vi "Facade.vi"(0 "Data In":T4, 2 "Display State In":T2, 3 "Container State":T3) -> (6 "Data Out":T4, 7 "Display State Out":T2, 8 "Action":T1)   [LabVIEW 2021, in "myRIO Choice Button.xctl"]
uses:
  <vilib>/myRIO/Common/Instrument Driver Framework/Utilities/xctls/myRIO Choice Button/myRIO Choice Button.xctl
  <vilib>/myRIO/Common/Instrument Driver Framework/Utilities/xctls/myRIO Choice Button/Data.ctl
  <vilib>/_xctls/Container State.ctl
  <vilib>/myRIO/Common/Instrument Driver Framework/Utilities/xctls/myRIO Choice Button/State.ctl
  <vilib>/_xctls/Action.ctl
  <vilib>/Utility/miscctls.llb/LVPositionTypeDef.ctl
  <vilib>/picture/picture.llb/imagedata.ctl
  <vilib>/_xctls/XControlSupport.lvlib
panel:
  out "Button Square":picture
  out "Explanation":string
  out "Title":string
  out "Glyph":picture
  out "Background":picture
types:
  T1 = typedef "XControlSupport.lvlib/Action.ctl" = cluster{"Data Changed?":bool, "State Changed?":bool, "Action Name":string}
  T2 = typedef "myRIO Choice Button.xctl/State.ctl" = cluster{"Title":string, "Explanation":string, "Mouse Enter Glyph":picture, "Mouse Down Glyph":picture, "Mouse Leave Glyph":picture, "Mouse Enter Background":picture, "Mouse Down Background":picture, "Mouse Leave Background":picture, "Button Mode":i32, "Button Square Frame":picture, "Disabled&GrayedOut":bool}
  T3 = typedef "XControlSupport.lvlib/Container State.ctl" = cluster{"Indicator?":bool, "Run Mode?":bool, " Refnum":refnum<vi>}
  T4 = typedef "myRIO Choice Button.xctl/Data.ctl" = bool
  T5 = typedef "LVPositionTypeDef.ctl" = cluster{"Left":i32, "Top":i32}
  T6 = enum8{"Enabled", "Disabled", "Disabled and Grayed Out"}
  T7 = typedef "imagedata.ctl" = cluster{"image type":i32, "image depth":i32, "image":u8[], "mask":u8[], "colors":u32[], "Rectangle":cluster{"left":i16, "top":i16, "right":i16, "bottom":i16}}
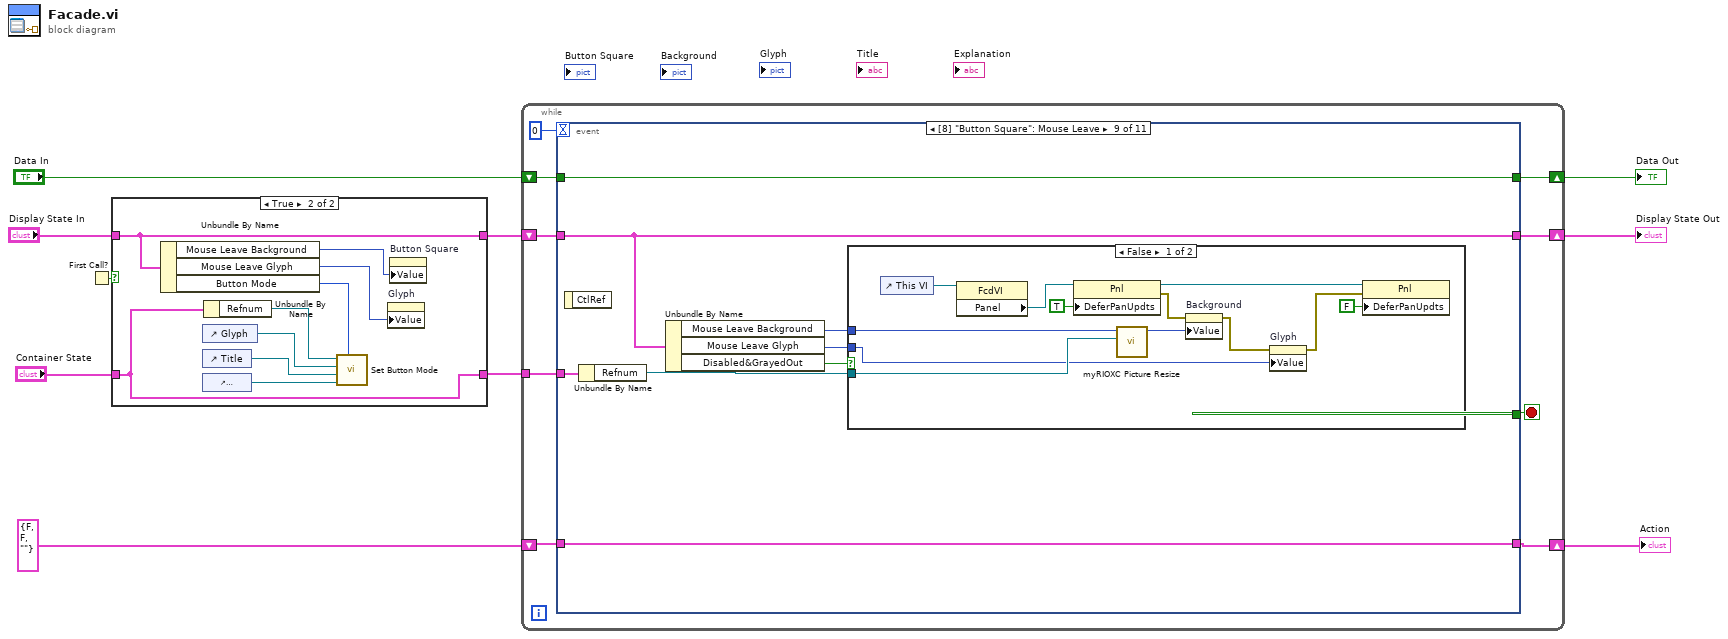
[diagram p0: block diagram]
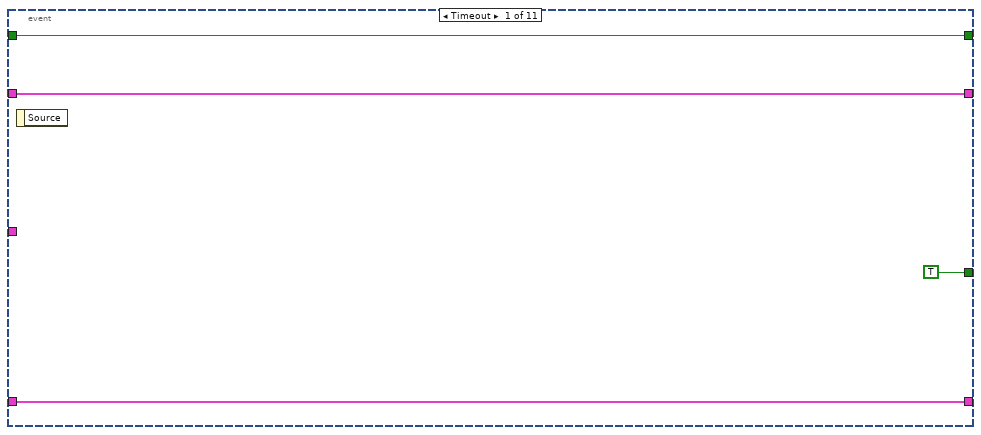
[diagram p3: hidden frame]
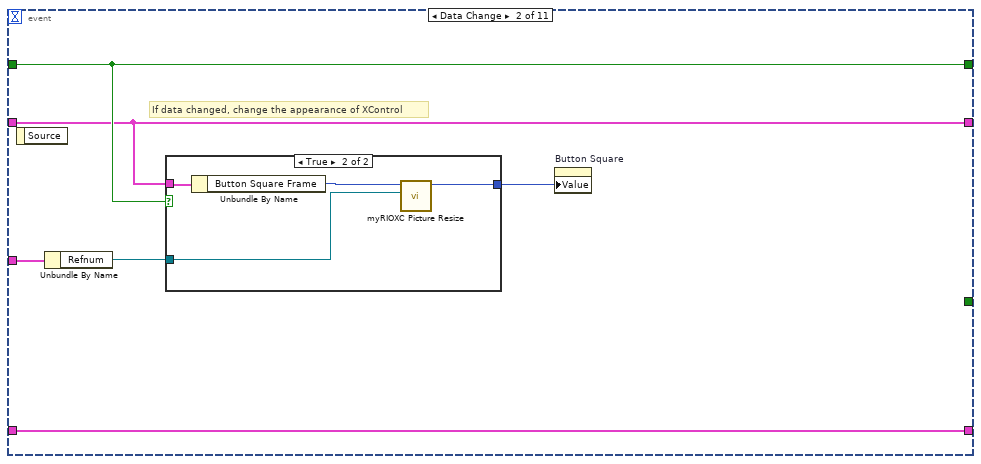
[diagram p4: hidden frame]
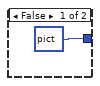
[diagram p5: hidden frame]
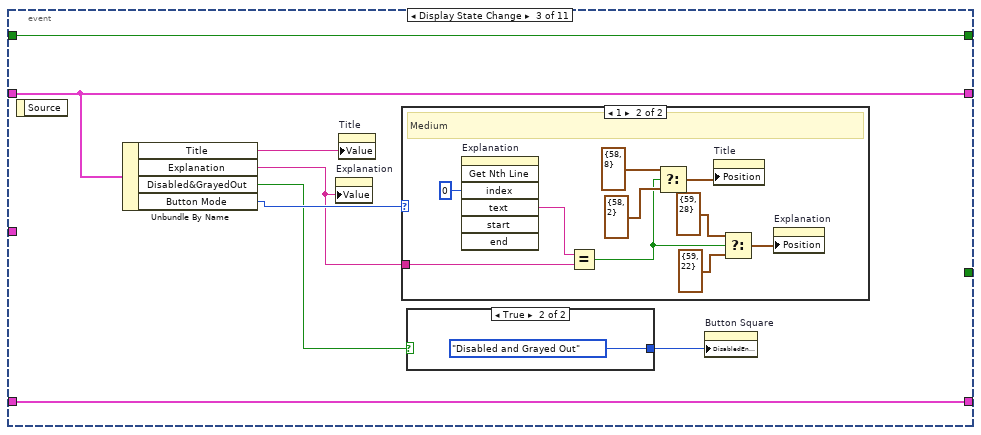
[diagram p6: hidden frame]
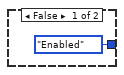
[diagram p8: hidden frame]
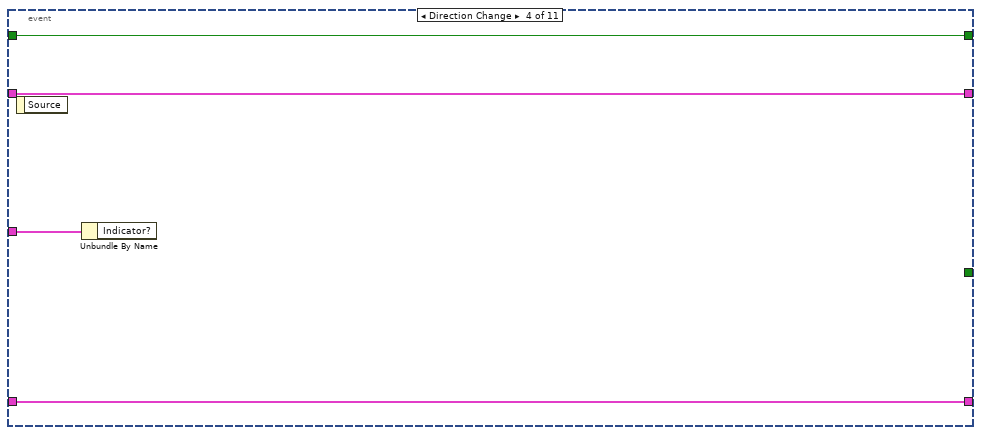
[diagram p9: hidden frame]
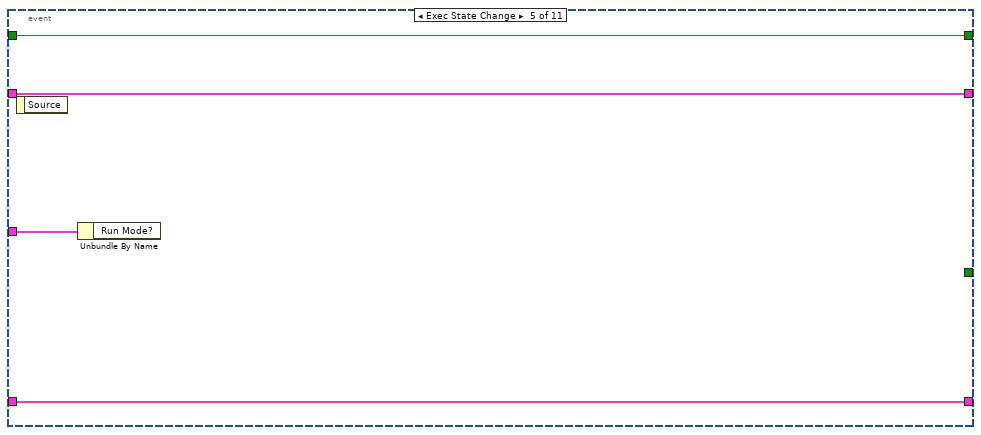
[diagram p10: hidden frame]
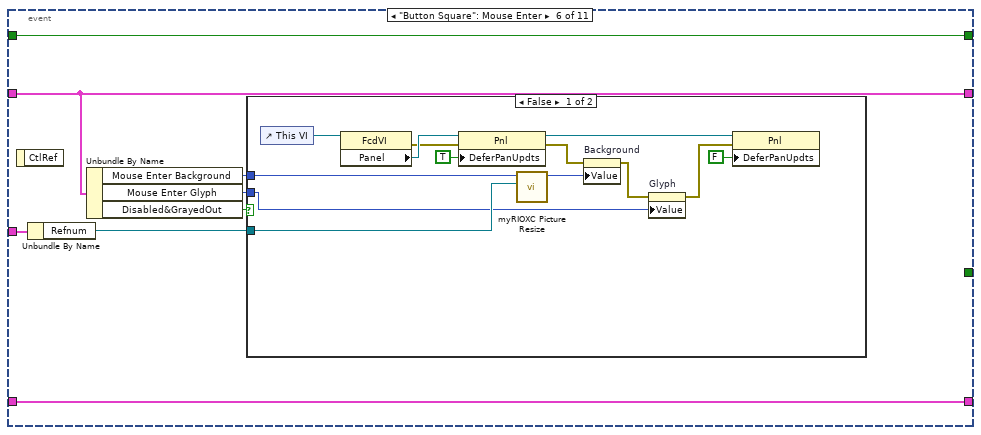
[diagram p11: hidden frame]
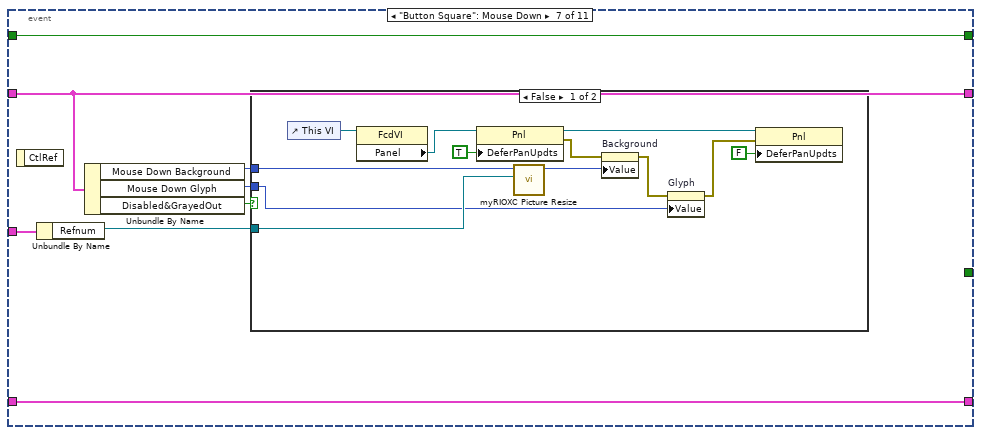
[diagram p13: hidden frame]
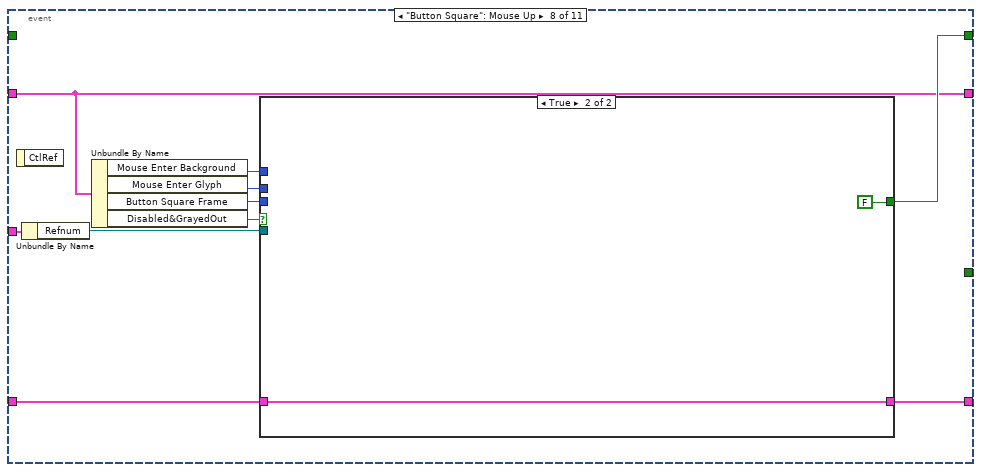
[diagram p15: hidden frame]
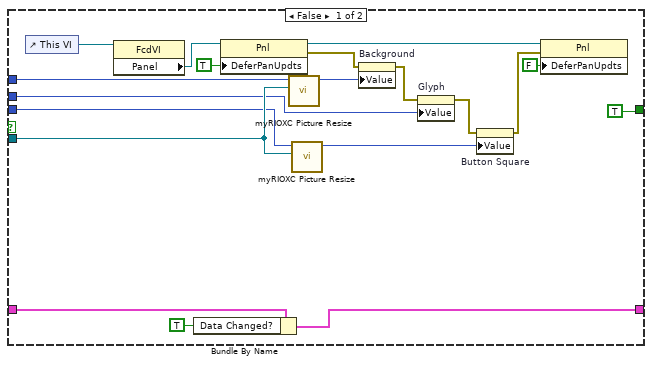
[diagram p16: hidden frame]
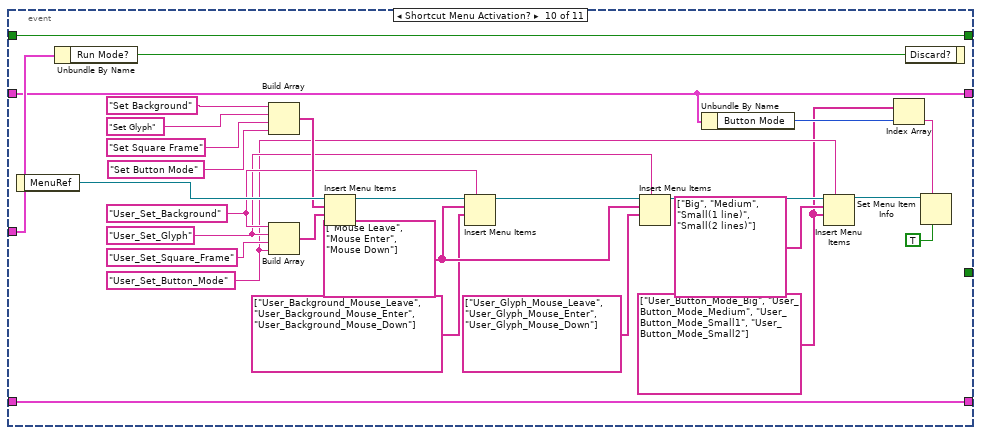
[diagram p18: hidden frame]
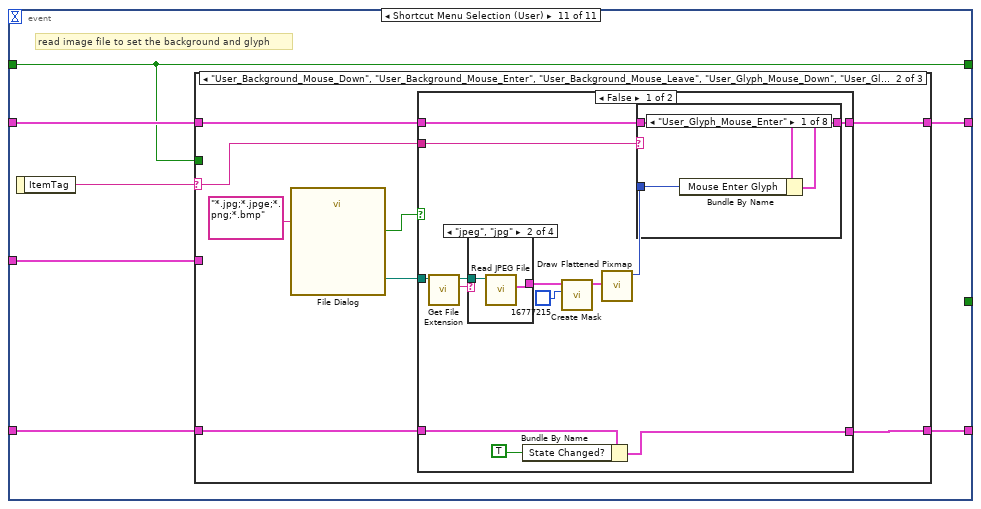
[diagram p19: hidden frame]
diagram:
  n1 = First Call?() -> (First Call?: T/F=w3:bool)
  n2 = case shown="True" w3 {
    tunnel: [w12 w19] -> w5
    tunnel: "Display State In" -> [w12 w19]
    tunnel: "Container State" -> [w11 w18]
    tunnel: [w11 w18] -> w1
    frame False {
    }
    frame True {
      n3 = Unbundle By Name(w19) -> ("Mouse Leave Background"=w20:picture, "Mouse Leave Glyph"=w21:picture, "Button Mode"=w17:i32)
      n4 = control-ref of="Glyph"() -> (w15:refnum<vi>)
      n5 = control-ref of="Title"() -> (w14:refnum<vi>)
      n6 = control-ref of="Explanation"() -> (w13:refnum<vi>)
      n7 = Unbundle By Name(w18) -> ("Refnum"=w16:refnum<vi>)
      n8 = call <vilib>:"Set Button Mode.vi"("Button Mode"=w17, "Explanation"=w13, "Title"=w14, "Glyph"=w15, "Container Reference"=w16) -> ()  [unwired: 7 in]
      n9 = property on="Glyph" class="Pict"("Value"=w21) -> ()  [unwired: 2 in, 2 out]
      n10 = property on="Button Square" class="Pict"("Value"=w20) -> ()  [unwired: 2 in, 2 out]
    }
  }
  n11 = while {
    shift-right: [w29] -> w8
    shift-left: w5 -> [w30]
    tunnel: w1 -> [w27]
    shift-right: [w25] -> w10
    shift-left: "Data In" -> [w26]
    shift-right: [w23] -> w7
    shift-left: T1 {"Data Changed?"=FALSE, "State Changed?"=FALSE, "Action Name"=""} ("Action") -> [w24]
    stop <- w28 stop-if-true
    n12 = event shown="[8] \"Button Square\": Mouse Leave" {
      selector: _ -> [_ _ _ _ _ _ _ _ _ _ _]
      dyn-events: _ -> [_ _ _ _ _ _ _ _ _ _ _]
      timeout: 0 -> [_ _ _ _ _ _ _ _ _ _ _]
      tunnel: w30 -> [w32 w37 w53 w68 w72 w77 w98 w120 w149 w171 w200]
      tunnel: [w32 w37 w53 w68 w72 w77 w98 w120 w149 w171 w199] -> w29
      tunnel: [TRUE _ _ _ _ _ _ _ _ _ _] -> w28
      tunnel: w27 -> [_ w36 _ w69 w73 w79 w100 w122 w151 w180 w195]
      tunnel: w26 -> [w31 w39 w50 w67 w71 w80 w101 _ w153 w193 w194]
      tunnel: [w31 w39 w50 w67 w71 w80 w101 w121 w153 w193 w194] -> w25
      tunnel: [w33 w40 w52 w66 w70 w81 w102 w123 w152 w192 w198] -> w23
      tunnel: w24 -> [w33 w40 w52 w66 w70 w81 w102 w124 w152 w192 w197]
      event Timeout {
        n13 = event-data() -> ()  [unwired: 1 in, 1 out]
      }
      event Data Change {
        # "If data changed, change the appearance of XControl"
        n14 = event-data() -> ()  [unwired: 1 in, 1 out]
        n15 = Unbundle By Name(w36) -> ("Refnum"=w35:refnum<vi>)
        n16 = case shown="True" w39 {
          tunnel: [picture data[5B] ("new picture") w43] -> w38
          tunnel: w37 -> [_ w45]
          tunnel: w35 -> [_ w42]
          frame False {
          }
          frame True {
            n17 = Unbundle By Name(w45) -> ("Button Square Frame"=w44:picture)
            n18 = call <vilib>:"myRIOXC Picture Resize.vi"("XCtrl Reference"=w42, "picture"=w44) -> ("new picture"=w43:picture)  [unwired: 9 in]
          }
        }
        n19 = property on="Button Square" class="Pict"("Value"=w38) -> ()  [unwired: 2 in, 2 out]
      }
      event Display State Change {
        n20 = event-data() -> ()  [unwired: 1 in, 1 out]
        n21 = Unbundle By Name(w53) -> ("Title"=w51:string, "Explanation"=w46:string, "Disabled&GrayedOut"=w47:bool, "Button Mode"=w48:i32)
        n22 = property on="Explanation" class="Str"("Value"=w46) -> ()  [unwired: 2 in, 2 out]
        n23 = property on="Title" class="Str"("Value"=w51) -> ()  [unwired: 2 in, 2 out]
        n24 = case shown="1" w48 {
          tunnel: w46 -> [_ w55]
          frame 0, Default {
            # "Other Modes"
          }
          frame 1 {
            # "Medium"
            n25 = invoke on="Explanation" class="Str" method="Get Nth Line"("index"=u32 0 ("line index")) -> ("text"=w56:string)  [unwired: 6 in, 6 out]
            n26 = Equal?(x=w56, y=w55) -> (x = y?=w54:bool)
            n27 = Select(t=T5 {"Left"=58, "Top"=8} ("Position"), s=w54, f=T5 {"Left"=58, "Top"=2}) -> (s? t:f=w62:T5)
            n28 = property on="Title" class="Str"("Position"=w62) -> ()  [unwired: 2 in, 2 out]
            n29 = Select(t=T5 {"Left"=59, "Top"=28} ("Position"), s=w54, f=T5 {"Left"=59, "Top"=22}) -> (s? t:f=w58:T5)
            n30 = property on="Explanation" class="Str"("Position"=w58) -> ()  [unwired: 2 in, 2 out]
          }
        }
        n31 = case shown="True" w47 {
          tunnel: [T6."Enabled" ("Disabled") T6."Disabled and Grayed Out" ("Disabled")] -> w49
          frame False {
          }
          frame True {
          }
        }
        n32 = property on="Button Square" class="Pict"("DisabledEnum"=w49) -> ()  [unwired: 2 in, 2 out]
      }
      event Direction Change {
        n33 = event-data() -> ()  [unwired: 1 in, 1 out]
        n34 = Unbundle By Name(w69) -> ()  [unwired: 1 out]
      }
      event Exec State Change {
        n35 = event-data() -> ()  [unwired: 1 in, 1 out]
        n36 = Unbundle By Name(w73) -> ()  [unwired: 1 out]
      }
      event "Button Square": Mouse Enter {
        n37 = event-data() -> ()  [unwired: 1 in, 1 out]
        n38 = Unbundle By Name(w79) -> ("Refnum"=w78:refnum<vi>)
        n39 = Unbundle By Name(w77) -> ("Mouse Enter Background"=w75:picture, "Mouse Enter Glyph"=w74:picture, "Disabled&GrayedOut"=w76:bool)
        n40 = case shown="False" w76 {
          tunnel: w78 -> [w93 _]
          tunnel: w75 -> [w83 _]
          tunnel: w74 -> [w82 _]
          frame False {
            n41 = control-ref of="This VI"() -> (w92:refnum<vi>)
            n42 = property class="FcdVI"(reference=w92) -> (error out=w90:errorcluster, "Panel"=w91:refnum<vi>)  [unwired: 1 in, 1 out]
            n43 = property class="Pnl"(reference=w91, error in=w90, "DeferPanUpdts"=TRUE ("Defer Panel Updates")) -> (reference out=w87:refnum<vi>, error out=w88:errorcluster)
            n44 = call <vilib>:"myRIOXC Picture Resize.vi"("XCtrl Reference"=w93, "picture"=w83) -> ("new picture"=w94:picture)  [unwired: 9 in]
            n45 = property on="Background" class="Pict"(error in=w88, "Value"=w94) -> (error out=w86:errorcluster)  [unwired: 1 in, 1 out]
            n46 = property on="Glyph" class="Pict"(error in=w86, "Value"=w82) -> (error out=w85:errorcluster)  [unwired: 1 in, 1 out]
            n47 = property class="Pnl"(reference=w87, error in=w85, "DeferPanUpdts"=FALSE ("Defer Panel Updates")) -> ()  [unwired: 2 out]
          }
          frame True {
          }
        }
      }
      event "Button Square": Mouse Down {
        n48 = event-data() -> ()  [unwired: 1 in, 1 out]
        n49 = Unbundle By Name(w100) -> ("Refnum"=w99:refnum<vi>)
        n50 = Unbundle By Name(w98) -> ("Mouse Down Background"=w95:picture, "Mouse Down Glyph"=w96:picture, "Disabled&GrayedOut"=w97:bool)
        n51 = case shown="False" w97 {
          tunnel: w99 -> [w113 _]
          tunnel: w96 -> [w104 _]
          tunnel: w95 -> [w103 _]
          frame False {
            n52 = control-ref of="This VI"() -> (w112:refnum<vi>)
            n53 = property class="FcdVI"(reference=w112) -> ("Panel"=w107:refnum<vi>)  [unwired: 1 in, 2 out]
            n54 = property class="Pnl"(reference=w107, "DeferPanUpdts"=TRUE ("Defer Panel Updates")) -> (reference out=w111:refnum<vi>, error out=w110:errorcluster)  [unwired: 1 in]
            n55 = call <vilib>:"myRIOXC Picture Resize.vi"("XCtrl Reference"=w113, "picture"=w103) -> ("new picture"=w114:picture)  [unwired: 9 in]
            n56 = property on="Background" class="Pict"(error in=w110, "Value"=w114) -> (error out=w109:errorcluster)  [unwired: 1 in, 1 out]
            n57 = property on="Glyph" class="Pict"(error in=w109, "Value"=w104) -> (error out=w108:errorcluster)  [unwired: 1 in, 1 out]
            n58 = property class="Pnl"(reference=w111, error in=w108, "DeferPanUpdts"=FALSE ("Defer Panel Updates")) -> ()  [unwired: 2 out]
          }
          frame True {
          }
        }
      }
      event "Button Square": Mouse Up {
        n59 = event-data() -> ()  [unwired: 1 in, 1 out]
        n60 = Unbundle By Name(w122) -> ("Refnum"=w119:refnum<vi>)
        n61 = Unbundle By Name(w120) -> ("Mouse Enter Background"=w117:picture, "Mouse Enter Glyph"=w116:picture, "Button Square Frame"=w115:picture, "Disabled&GrayedOut"=w118:bool)
        n62 = case shown="True" w118 {
          tunnel: w124 -> [w143 w145]
          tunnel: [w142 w145] -> w123
          tunnel: [T4 TRUE ("Data In") T4 FALSE ("Data In")] -> w121
          tunnel: w119 -> [w137 _]
          tunnel: w117 -> [w127 _]
          tunnel: w116 -> [w126 _]
          tunnel: w115 -> [w125 _]
          frame False {
            n63 = control-ref of="This VI"() -> (w132:refnum<vi>)
            n64 = property class="FcdVI"(reference=w132) -> ("Panel"=w133:refnum<vi>)  [unwired: 1 in, 2 out]
            n65 = Bundle By Name(cluster=w143, "Data Changed?"=TRUE) -> (w142:T1)
            n66 = property class="Pnl"(reference=w133, "DeferPanUpdts"=TRUE ("Defer Panel Updates")) -> (reference out=w135:refnum<vi>, error out=w131:errorcluster)  [unwired: 1 in]
            n67 = call <vilib>:"myRIOXC Picture Resize.vi"("XCtrl Reference"=w137, "picture"=w127) -> ("new picture"=w139:picture)  [unwired: 9 in]
            n68 = call <vilib>:"myRIOXC Picture Resize.vi"("XCtrl Reference"=w137, "picture"=w125) -> ("new picture"=w138:picture)  [unwired: 9 in]
            n69 = property on="Background" class="Pict"(error in=w131, "Value"=w139) -> (error out=w130:errorcluster)  [unwired: 1 in, 1 out]
            n70 = property on="Glyph" class="Pict"(error in=w130, "Value"=w126) -> (error out=w129:errorcluster)  [unwired: 1 in, 1 out]
            n71 = property on="Button Square" class="Pict"(error in=w129, "Value"=w138) -> (error out=w128:errorcluster)  [unwired: 1 in, 1 out]
            n72 = property class="Pnl"(reference=w135, error in=w128, "DeferPanUpdts"=FALSE ("Defer Panel Updates")) -> ()  [unwired: 2 out]
          }
          frame True {
          }
        }
      }
      event "Button Square": Mouse Leave {
        n73 = event-data() -> ()  [unwired: 1 in, 1 out]
        n74 = Unbundle By Name(w151) -> ("Refnum"=w150:refnum<vi>)
        n75 = Unbundle By Name(w149) -> ("Mouse Leave Background"=w148:picture, "Mouse Leave Glyph"=w147:picture, "Disabled&GrayedOut"=w146:bool)
        n76 = case shown="False" w146 {
          tunnel: w150 -> [w164 _]
          tunnel: w148 -> [w155 _]
          tunnel: w147 -> [w154 _]
          frame False {
            n77 = control-ref of="This VI"() -> (w161:refnum<vi>)
            n78 = property class="FcdVI"(reference=w161) -> ("Panel"=w160:refnum<vi>)  [unwired: 1 in, 2 out]
            n79 = property class="Pnl"(reference=w160, "DeferPanUpdts"=TRUE ("Defer Panel Updates")) -> (reference out=w159:refnum<vi>, error out=w158:errorcluster)  [unwired: 1 in]
            n80 = call <vilib>:"myRIOXC Picture Resize.vi"("XCtrl Reference"=w164, "picture"=w155) -> ("new picture"=w165:picture)  [unwired: 9 in]
            n81 = property on="Background" class="Pict"(error in=w158, "Value"=w165) -> (error out=w157:errorcluster)  [unwired: 1 in, 1 out]
            n82 = property on="Glyph" class="Pict"(error in=w157, "Value"=w154) -> (error out=w156:errorcluster)  [unwired: 1 in, 1 out]
            n83 = property class="Pnl"(reference=w159, error in=w156, "DeferPanUpdts"=FALSE ("Defer Panel Updates")) -> ()  [unwired: 2 out]
          }
          frame True {
          }
        }
      }
      event Shortcut Menu Activation? {
        w166 = string[] ["User_Button_Mode_Big", "User_Button_Mode_Medium", "User_Button_Mode_Small1", "User_Button_Mode_Small2"] ("item tags")
        w173 = "User_Set_Button_Mode"
        w181 = "User_Set_Glyph"
        w182 = "User_Set_Background"
        w186 = string[] ["Mouse Leave", "Mouse Enter", "Mouse Down"] ("item tags")
        n84 = event-data() -> ("MenuRef"=w191:refnum<k9>)  [unwired: 1 in]
        n85 = Unbundle By Name(w180) -> ("Run Mode?"=w179:bool)
        n86 = Build Array("Set Background" ("menu tag"), "Set Glyph" ("menu tag"), "Set Square Frame" ("menu tag"), "Set Button Mode" ("menu tag")) -> (w187:string[])
        n87 = Build Array(w182, w181, "User_Set_Square_Frame", w173) -> (w183:string[])
        n88 = Insert Menu Items(7:w183, 8:w187, 9:w191) -> (3:w178:refnum<k9>)  [unwired: 3 in, 2 out]
        n89 = Insert Menu Items(5:w182, 7:string[] ["User_Background_Mouse_Leave", "User_Background_Mouse_Enter", "User_Background_Mouse_Down"] ("item tags"), 8:w186, 9:w178) -> (3:w190:refnum<k9>)  [unwired: 2 in, 2 out]
        n90 = Insert Menu Items(5:w181, 7:string[] ["User_Glyph_Mouse_Leave", "User_Glyph_Mouse_Enter", "User_Glyph_Mouse_Down"] ("item tags"), 8:w186, 9:w190) -> (3:w174:refnum<k9>)  [unwired: 2 in, 2 out]
        n91 = Unbundle By Name(w171) -> ("Button Mode"=w169:i32)
        n92 = Insert Menu Items(5:w173, 7:w166, 8:string[] ["Big", "Medium", "Small(1 line)", "Small(2 lines)"] ("item tags"), 9:w174) -> (3:w172:refnum<k9>)  [unwired: 2 in, 2 out]
        n93 = Index Array(array=w166, index=w169) -> (element=w168:string)
        n94 = event-data("Discard?"=w179) -> ()  [unwired: 1 in, 1 out]
        n95 = Set Menu Item Info(6:TRUE ("checked"), 7:w168, 11:w172) -> ()  [unwired: 4 in, 2 out]
      }
      event Shortcut Menu Selection (User) {
        # "read image file to set the background and glyph"
        n96 = event-data() -> ("ItemTag"=w196:string)  [unwired: 1 in]
        n97 = case shown="\"User_Background_Mouse_Down\", \"User_Background_Mouse_Enter\", \"User_Background_Mouse_Leave\", \"User_Glyph_Mouse_Down\", \"User_Glyph_Mouse_Enter\", \"User_Glyph_Mouse_Leave\", \"User_Set_Square_Frame\"" w196 {
          selector: w196 -> [_ w203 w258]
          tunnel: w200 -> [w202 w210 w256]
          tunnel: [w202 w209 w262] -> w199
          tunnel: [w201 w208 w265] -> w198
          tunnel: w197 -> [w201 w207 w266]
          tunnel: w195 -> [_ _ w263]
          tunnel: w194 -> [_ _ _]
          frame Default {
          }
          frame "User_Background_Mouse_Down", "User_Background_Mouse_Enter", "User_Background_Mouse_Leave", "User_Glyph_Mouse_Down", "User_Glyph_Mouse_Enter", "User_Glyph_Mouse_Leave", "User_Set_Square_Frame" {
            n98 = call "File Dialog"("pattern (all files)"="*.jpg;*.jpge;*.png;*.bmp") -> ("selected path"=w205:path, "cancelled"=w204:bool)  [unwired: 11 in, 2 out]
            n99 = case shown="False" w204 {
              tunnel: w203 -> [w223 _]
              tunnel: w210 -> [w222 w254]
              tunnel: [w221 w254] -> w209
              tunnel: [w220 w253] -> w208
              tunnel: w207 -> [w218 w253]
              tunnel: w205 -> [w217 _]
              frame False {
                n100 = call <vilib>:"Get File Extension.vi"("file"=w217) -> ("lowercase file extension"=w216:string, "dup file"=w215:path)  [unwired: 6 in, 3 out]
                n101 = case shown="\"jpeg\", \"jpg\"" w216 {
                  tunnel: w215 -> [w225 w227 _ w230]
                  tunnel: [w224 w226 T7 {"image type"=0, "image depth"=0, "image"=[], "mask"=[], "colors"=[], "Rectangle"={"left"=0, "top"=0, "right"=0, "bottom"=0}} ("image data") w229] -> w212
                  frame "bmp" {
                    n102 = call <vilib>:"Read BMP File.vi"("path to BMP file"=w225) -> ("image data"=w224:T7)  [unwired: 8 in, 2 out]
                  }
                  frame "jpeg", "jpg" {
                    n103 = call <vilib>:"Read JPEG File.vi"("path to JPEG file"=w227) -> ("image data"=w226:T7)  [unwired: 8 in, 2 out]
                  }
                  frame Default {
                  }
                  frame "png" {
                    n104 = call <vilib>:"Read PNG File.vi"("path to PNG file"=w230) -> ("image data"=w229:T7)  [unwired: 8 in, 2 out]
                  }
                }
                n105 = Bundle By Name(cluster=w218, "State Changed?"=TRUE) -> (w220:T1)
                n106 = call <vilib>:"Create Mask.vi"("Mask Color (Black)"=u32 16777215, "image data"=w212) -> ("image data"=w211:T7)  [unwired: 9 in]
                n107 = call <vilib>:"Draw Flattened Pixmap.vi"("image data"=w211) -> ("new picture"=w214:picture)  [unwired: 8 in]
                n108 = case shown="\"User_Glyph_Mouse_Enter\"" w223 {
                  tunnel: w222 -> [w232 w234 w237 w240 w243 w246 w249 w252]
                  tunnel: [w233 w234 w236 w239 w242 w245 w248 w251] -> w221
                  tunnel: w214 -> [w231 _ w235 w238 w241 w244 w247 w250]
                  frame "User_Glyph_Mouse_Enter" {
                    n109 = Bundle By Name(cluster=w232, "Mouse Enter Glyph"=w231) -> (w233:T2)
                  }
                  frame Default {
                  }
                  frame "User_Background_Mouse_Enter" {
                    n110 = Bundle By Name(cluster=w237, "Mouse Enter Background"=w235) -> (w236:T2)
                  }
                  frame "User_Background_Mouse_Down" {
                    n111 = Bundle By Name(cluster=w240, "Mouse Down Background"=w238) -> (w239:T2)
                  }
                  frame "User_Background_Mouse_Leave" {
                    n112 = Bundle By Name(cluster=w243, "Mouse Leave Background"=w241) -> (w242:T2)
                  }
                  frame "User_Glyph_Mouse_Down" {
                    n113 = Bundle By Name(cluster=w246, "Mouse Down Glyph"=w244) -> (w245:T2)
                  }
                  frame "User_Glyph_Mouse_Leave" {
                    n114 = Bundle By Name(cluster=w249, "Mouse Leave Glyph"=w247) -> (w248:T2)
                  }
                  frame "User_Set_Square_Frame" {
                    n115 = Bundle By Name(cluster=w252, "Button Square Frame"=w250) -> (w251:T2)
                  }
                }
              }
              frame True {
              }
            }
          }
          frame "User_Button_Mode_Big", "User_Button_Mode_Medium", "User_Button_Mode_Small1", "User_Button_Mode_Small2" {
            n116 = Unbundle By Name(w263) -> ("Refnum"=w255:refnum<vi>)
            n117 = case shown="\"User_Button_Mode_Medium\"" w258 {
              tunnel: [0 1 2 3] -> w257
              frame "User_Button_Mode_Big", Default {
              }
              frame "User_Button_Mode_Medium" {
              }
              frame "User_Button_Mode_Small1" {
              }
              frame "User_Button_Mode_Small2" {
              }
            }
            n118 = Bundle By Name(cluster=w266, "State Changed?"=TRUE ("Data Changed?")) -> (w265:T1)
            n119 = control-ref of="Glyph"() -> (w261:refnum<vi>)
            n120 = control-ref of="Title"() -> (w260:refnum<vi>)
            n121 = control-ref of="Explanation"() -> (w259:refnum<vi>)
            n122 = call <vilib>:"Set Button Mode.vi"("Button Mode"=w257, "Explanation"=w259, "Title"=w260, "Glyph"=w261, "Container Reference"=w255) -> ()  [unwired: 7 in]
            n123 = Bundle By Name(cluster=w256, "Button Mode"=w257) -> (w262:T2)
          }
        }
      }
    }
  }
  "Display State Out" <- w8
  "Data Out" <- w10
  "Action" <- w7
